vi "AH_msgTEST.vi"() -> ()   [LabVIEW 2021]
uses:
  AH_CmdSRE.vi
  Measurement_Cluster.ctl
  Data_Cluster.ctl
  Mode_Enum.ctl
  Config_Cluster.ctl
panel:
  in  "Configuration Cluster":T1={"General"={"Config.ini"=path "", "Default Logging Path"=path ""}, "Hardware"={"Measure Rate (1/s)"=0, "HP DMM VISA"="", "LS 335 VISA"=""}, "Operation"={"Operation Mode"=enum."Idle-Off", "Status"="", "NewLog?"=FALSE, "OvenWarn"=FALSE}}
  in  "Data Cluster In":T3 {"GUI Data Cluster"."SBR" format="%08b"}
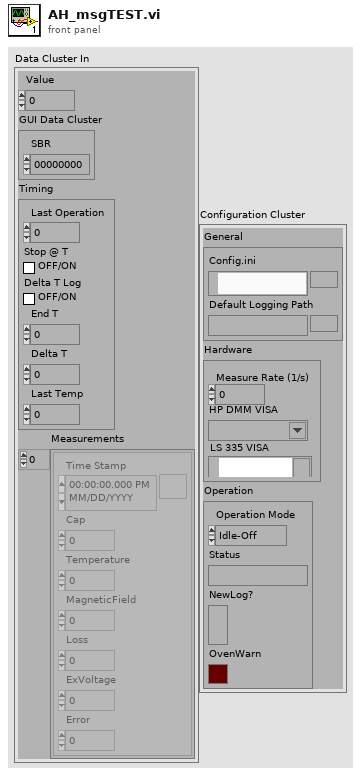
[diagram p1: front panel]
types:
  T1 = typedef "Config_Cluster.ctl" = cluster{"General":cluster{"Config.ini":path, "Default Logging Path":path}, "Hardware":cluster{"Measure Rate (1/s)":i32, "HP DMM VISA":refnum<visa-resource-name>, "LS 335 VISA":refnum<visa-resource-name>}, "Operation":cluster{"Operation Mode":T2, "Status":string, "NewLog?":bool, "OvenWarn":bool}}
  T2 = typedef "Mode_Enum.ctl" = enum16{"OvenNRDY", "Logging", "Idle-Off", "Idle"}
  T3 = typedef "Data_Cluster.ctl" = cluster{"Value":dbl, "GUI Data Cluster":cluster{"SBR":u16}, "Timing":cluster{"Last Operation":dbl, "Stop @ T":bool, "Delta T Log":bool, "End T":dbl, "Delta T":dbl, "Last Temp":dbl}, "Measurements":T4[]}
  T4 = typedef "Measurement_Cluster.ctl" = cluster{"Time Stamp":timestamp, "Cap":dbl, "Temperature":dbl, "MagneticField":dbl, "Loss":dbl, "ExVoltage":dbl, "Error":dbl}
  T5 = typedef "Config_Cluster.ctl" = cluster{"General":cluster{"Config.ini":path, "Default Logging Path":path}, "Hardware":cluster{"AHC VISA COM":refnum<visa-resource-name>, "Measure Rate (1/s)":i32, "Global T VAR":refnum<k21>, "Global B VAR":refnum<k21>, "Average":u8, "Bias":u8, "Cable":cluster{"Length":dbl, "Resistance":dbl, "Inductance":dbl, "Capacitance":dbl}, "Tracking":u8, "Voltage":dbl}, "Operation":cluster{"Operation Mode":T2, "Status":string, "NewLog?":bool, "OvenWarn":bool}}
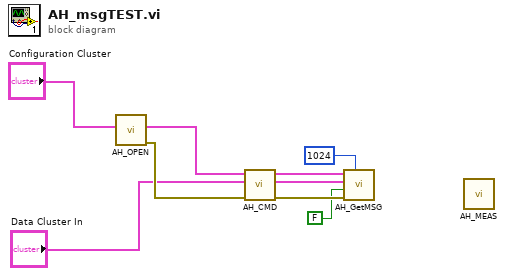
[diagram p0: block diagram]
diagram:
  n1 = call "AH_OPEN.vi"("Configuration Cluster"="Configuration Cluster") -> ("error out"=w8:errorcluster, "Configuration Cluster Out"=w9:T1)  [unwired: 9 in]
  n2 = call-poly "AH_CMD.vi"("error in (no error)"=w8, "Data Cluster In"="Data Cluster In", "Config Cluster In"=w9) -> ("error IO"=w3:errorcluster, "Data Cluster Out"=w4:T3, "Configuration Cluster Out"=w5:T5)  [unwired: 6 in]
  n3 = call "AH_GetMSG.vi"("byte count"=u32 1024, "error in (no error)"=w3, "Halt For RQS"=FALSE, "Data Cluster In"=w4, "Config Cluster In"=w5) -> ()  [unwired: 1 in, 6 out]
  n4 = call "AH_MEAS.vi"() -> ()  [unwired: 7 in, 9 out]
